vi "Accelerometer.vi"() -> ()   [LabVIEW 2012]
uses:
  <vilib>/LabVIEW Targets/FPGA/cRIO/shared/nicrio_ModuleControls/nicrio_cRIO-9234_DataRatesRing2.ctl
  <vilib>/rvi/Emulation/niFpgaSctlEmulationGetInTimedLoop.vi
  <vilib>/rvi/Emulation/niFpgaSctlEmulationGlobalWrite.vi
  <vilib>/rvi/eio/common/nirviEmuTemplatePropertySet_noerrors.vi
  <vilib>/rvi/FIFO/Fifo_Resource/nirvififoEmulationSetSize.vi
  <vilib>/rvi/DataTransferAndStorage/Container/Common/niFpgaContainerGetUniqueNameForEmu.vi
  <vilib>/rvi/eio/common/nirviEmuTemplateMethod_errors.vi
  <vilib>/rvi/Emulation/niFpgaSctlEmulationFifoFullMgr.vi
  <vilib>/rvi/errors/niFpgaSetErrorForExecOnDevCompSimple.vi
  <vilib>/rvi/eio/common/nirviEmuReportErrorAndStop.vi
  <vilib>/rvi/Emulation/niFpgaSctlEmulationResourceMgr.vi
  <vilib>/eio/EIOPropertyNode/EIOPropertyNode.xnode
  <vilib>/rvi/DataTransferAndStorage/Container/XNode/niFpgaContainer.xnode
  <vilib>/rvi/FIFO/Fifo_Resource/nirvififoEmulationClear.vi
  <vilib>/eio/EIONode/EIONode.xnode
  <vilib>/rvi/FIFO/Fifo_Resource/nirvififoEmulationRead.vi
  <vilib>/rvi/FIFO/Fifo_Resource/nirvififoEmulationWrite.vi
  <vilib>/rvi/eio/common/nirviEmuTemplatePropertyGet_errors.vi
  <vilib>/rvi/eio/common/nirviEmuTemplatePropertyGet_noerrors.vi
  <vilib>/rvi/eio/common/nirviEmuTemplatePropertySet_errors.vi
panel:
  out "Y Acceleration":fxp<+/-,24,4>
  in  "Data Rate":T1=1 items=["51.200 kS/s (NI 9234)"=1, "25.600 kS/s (NI 9234)"=2, "17.067 kS/s (NI 9234)"=3, "12.800 kS/s (NI 9234)"=4, "10.240 kS/s (NI 9234)"=5, "8.533 kS/s (NI 9234)"=6, "7.314 kS/s (NI 9234)"=7, "6.400 kS/s (NI 9234)"=8, "5.689 kS/s (NI 9234)"=9, "5.120 kS/s (NI 9234)"=10, "4.654 kS/s (NI 9234)"=11, "4.267 kS/s (NI 9234)"=12, "3.938 kS/s (NI 9234)"=13, "3.657 kS/s (NI 9234)"=14, "3.413 kS/s (NI 9234)"=15, "3.200 kS/s (NI 9234)"=16, "3.012 kS/s (NI 9234)"=17, "2.845 kS/s (NI 9234)"=18, "2.695 kS/s (NI 9234)"=19, "2.560 kS/s (NI 9234)"=20, "2.438 kS/s (NI 9234)"=21, "2.328 kS/s (NI 9234)"=22, "2.226 kS/s (NI 9234)"=23, "2.133 kS/s (NI 9234)"=24, "2.048 kS/s (NI 9234)"=25, "1.969 kS/s (NI 9234)"=26, "1.896 kS/s (NI 9234)"=27, "1.829 kS/s (NI 9234)"=28, "1.765 kS/s (NI 9234)"=29, "1.707 kS/s (NI 9234)"=30, "1.652 kS/s (NI 9234)"=31]
  out "Terminate":bool
  in  "Acceleration Threshold":fxp<+/-,24,4> format="%.22g"
  in  "Fan Speed Control":fxp<+/-,20,5> format="%_6g"
  out "Threshold Exceeded?":bool
  in  "Stop":bool
  out "Overflow Occurred?":bool
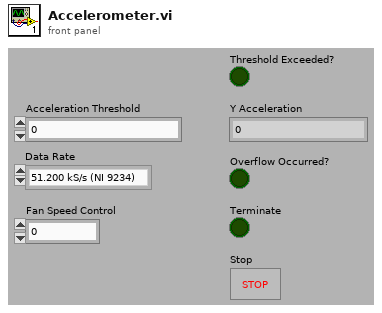
[diagram p1: front panel]
types:
  T1 = typedef "nicrio_cRIO-9234_DataRatesRing2.ctl" = u8
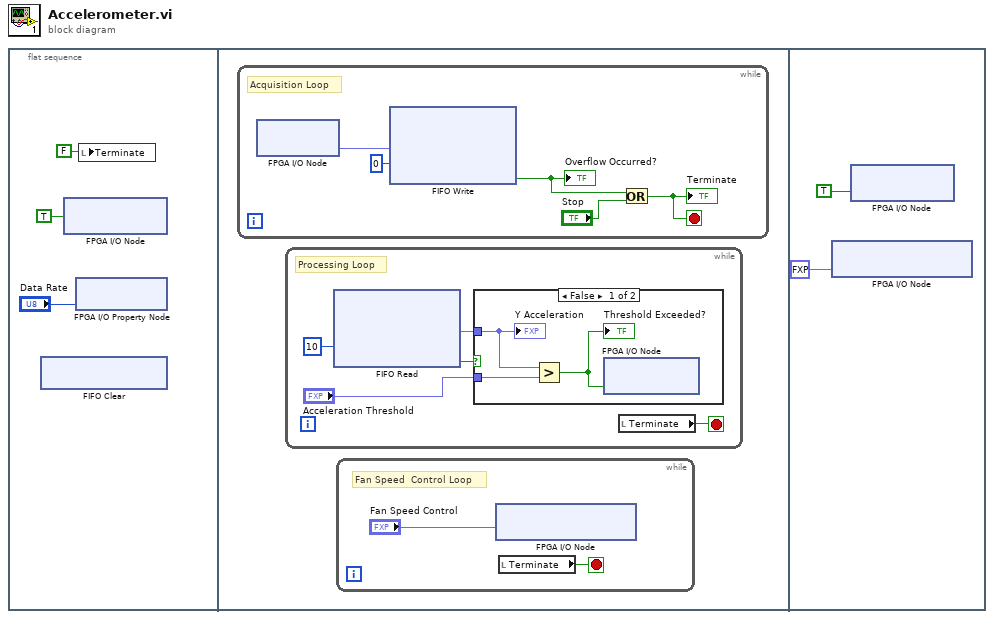
[diagram p0: block diagram]
diagram:
  n1 = flat-sequence {
    frame #0 {
      n2 = xnode "FIFO Clear"() -> ()  [unwired: 1 in, 1 out]
      n3 = xnode "FPGA I/O Node"("Mod2/Start"=TRUE) -> ()  [unwired: 1 in, 1 out]
      n4 = xnode "FPGA I/O Property Node"("Data Rate"="Data Rate") -> ()  [unwired: 1 in, 1 out]
      n5 = local write "Terminate"(FALSE ("Terminate 2")) -> ()
    }
    frame #1 {
      n6 = while {
        stop <- w16 stop-if-true
        # "Acquisition Loop"
        n7 = xnode "FPGA I/O Node"() -> ("Y Accel"=w14:fxp<+/-,24,4>)  [unwired: 1 in, 1 out]
        n8 = xnode "FIFO Write"("Element"=w14, "Timeout"=0) -> ("Timed Out?"=w17:bool)  [unwired: 1 in, 1 out]
        "Overflow Occurred?" <- w17
        n9 = Or(x=w17, y="Stop") -> (x .or. y?=w16:bool)
        "Terminate" <- w16
      }
      n10 = while {
        stop <- w10 stop-if-true
        # "Processing Loop"
        n11 = xnode "FIFO Read"("Timeout"=10) -> ("Element"=w8:fxp<+/-,24,4>, "Timed Out?"=w7:bool)  [unwired: 1 in, 1 out]
        n12 = case shown="False" w7 {
          tunnel: w8 -> [w12 _]
          tunnel: "Acceleration Threshold" -> [w11 _]
          frame False {
            n13 = Greater?(x=w12, y=w11) -> (0:w13:bool)
            "Threshold Exceeded?" <- w13
            n14 = xnode "FPGA I/O Node"("FPGA LED"=w13) -> ()  [unwired: 1 in, 1 out]
            "Y Acceleration" <- w12
          }
          frame True {
          }
        }
        n15 = local read "Terminate"() -> (w10:bool)
      }
      n16 = while {
        stop <- w5 stop-if-true
        # "Fan Speed  Control Loop"
        n17 = xnode "FPGA I/O Node"("Fan Speed Control"="Fan Speed Control") -> ()  [unwired: 1 in, 1 out]
        n18 = local read "Terminate"() -> (w5:bool)
      }
    }
    frame #2 {
      n19 = xnode "FPGA I/O Node"("Fan Speed Control"=fxp<+/-,20,5> 0.0) -> ()  [unwired: 1 in, 1 out]
      n20 = xnode "FPGA I/O Node"("Mod2/Stop"=TRUE ("Mod2/Start")) -> ()  [unwired: 1 in, 1 out]
    }
  }
